vi "transfer file to sd card.vi"(7 "output number":u8=1 min=1 max=2, 8 "error in":errorcluster, 9 "disk file name":string, 10 "input file":path, 11 "Teensy Serial Port":refnum<visa-resource-name>) -> (0 "error out":errorcluster, 3 "teensy serial port out":refnum<visa-resource-name>, 4 "commands and responses":string)   [LabVIEW 2013]
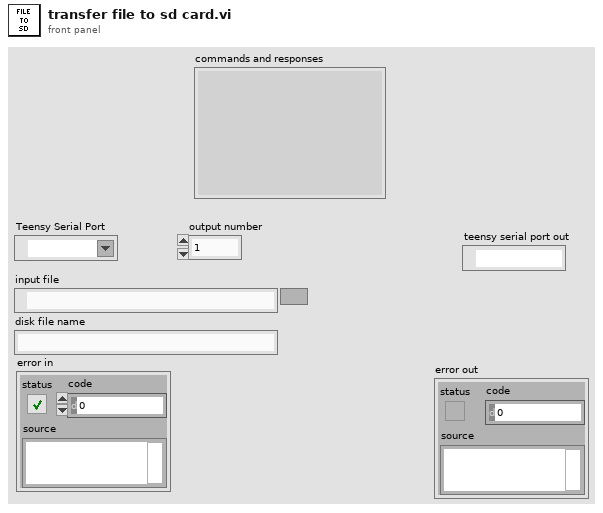
[diagram p1: front panel]
types:
  T1 = enum16{"R - open file for Reading", "W - open file for Writing", "S - send bytes", "F - fetch bytes", "B - begin experiment", "E - end experiment", "N - set number of bits per frame", "I - get info", "Q - Quiet (only error msgs)", "L - Loud (acknowledge all)", "T - set stimulus state", "Y - ready to start experiment", "H - useless Help message", "C - Close file", "O - enable/disable output"}
  T2 = enum16{"big-endian, network order", "native, host order", "little-endian"}
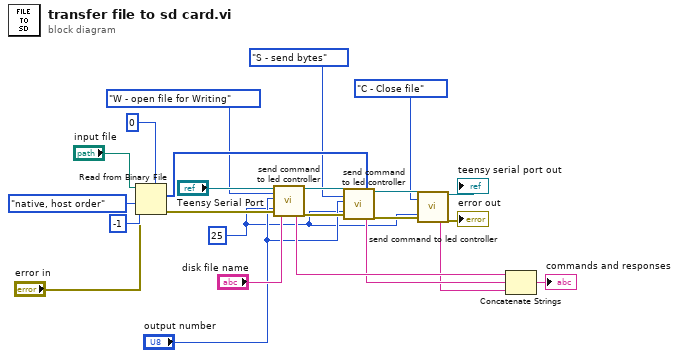
[diagram p0: block diagram]
diagram:
  w4 = u32 25 ("milliseconds to wait between write and read")
  n1 = Read from Binary File(5:u8 0 ("count (1)"), 8:"error in", 9:T2."native, host order" ("byte order (0:big-endian, network order)"), 10:-1 ("count (1)"), 11:"input file") -> (0:w20:errorcluster, 2:w17:u8[])  [unwired: 1 in, 2 out]
  n2 = call "send command to led controller.vi"("Teensy Serial Port"="Teensy Serial Port", "Command"=T1."W - open file for Writing", "lednumber"="output number", "milliseconds to wait between write and read"=w4, "error in"=w20, "file name"="disk file name") -> ("command and response with time"=w9:string, "teensy serial port out"=w12:refnum<visa-resource-name>, "error out"=w18:errorcluster)  [unwired: 8 in, 3 out]
  n3 = call "send command to led controller.vi"("Teensy Serial Port"=w12, "Command"=T1."S - send bytes", "lednumber"="output number", "milliseconds to wait between write and read"=w4, "error in"=w18, "bytes to send"=w17) -> ("command and response with time"=w8:string, "teensy serial port out"=w11:refnum<visa-resource-name>, "error out"=w16:errorcluster)  [unwired: 8 in, 3 out]
  n4 = call "send command to led controller.vi"("Teensy Serial Port"=w11, "Command"=T1."C - Close file", "milliseconds to wait between write and read"=w4, "error in"=w16) -> ("command and response with time"=w7:string, "teensy serial port out"=→"teensy serial port out":refnum<visa-resource-name>, "error out"=→"error out":errorcluster)  [unwired: 10 in, 3 out]
  n5 = Concatenate Strings(w9, w8, w7) -> (→"commands and responses":string)
